vi "leak_tester_0.vi"() -> ()   [LabVIEW 2020]
uses:
  event_controller.ctl
  <vilib>/Spiers New Technologies/SNT/Alfred-Connector/Utilities/Parse Item Label Data Output.ctl
  <vilib>/Spiers New Technologies/SNT/Alfred-Connector/Alfred.lvlib
panel:
  in  "RETURN":bool
  in  "test":bool
  out "Parse Item Label Data out":T1
  out "result":bool
  in  "Barcode":string="IID:287454SN:CM5810B759GBRED11031550695872PN:CM5810B759GBEND"
  out "User ID":string
  out "Enum":T2
  in  "Badge":string="3B 88 01 00 03 08 06 66 00 77 80 78"
  in  "enter":bool
  in  "stop":bool
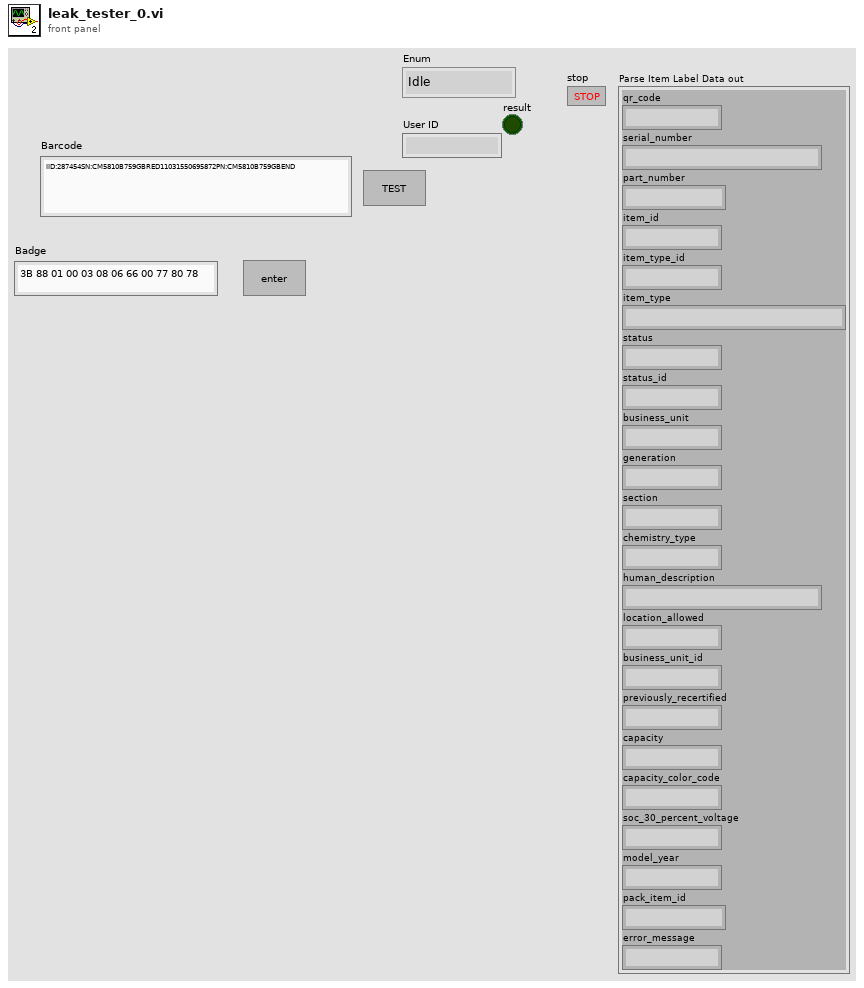
[diagram p1: front panel]
types:
  T1 = typedef "Alfred.lvlib/Parse Item Label Data Output.ctl" = cluster{"qr_code":string, "serial_number":string, "part_number":string, "item_id":string, "item_type_id":string, "item_type":string, "status":string, "status_id":string, "business_unit":string, "generation":string, "section":string, "chemistry_type":string, "human_description":string, "location_allowed":string, "business_unit_id":string, "previously_recertified":string, "capacity":string, "capacity_color_code":string, "soc_30_percent_voltage":string, "model_year":string, "pack_item_id":string, "error_message":string}
  T2 = typedef "event_controller.ctl" = enum16{"Idle", "LoginFalse", "BatteryScan", "BatteryError", "Testing", "Submission"}
  T3 = cluster{"item_id":string, "item_type_id":string, string}
  T4 = cluster{"Username":string, "Badge":string, "Username":string, "Privilege":string}
  T5 = typedef "Alfred.lvlib/Login Info Return.ctl" = cluster{"User ID":string, "Username":string, "First Name":string, "Last Name":string, "E-mail":string, "Time Zone":string, "Error Message":string}
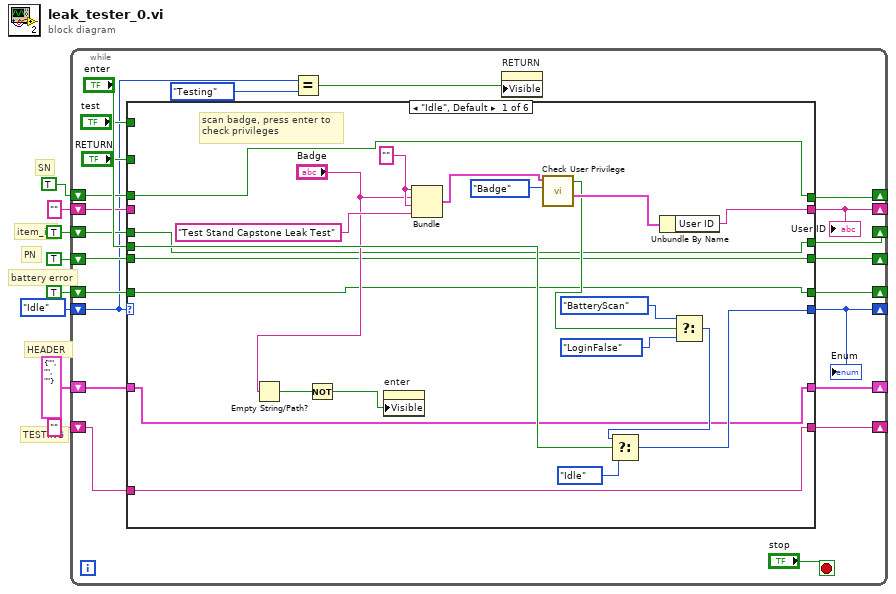
[diagram p0: block diagram]
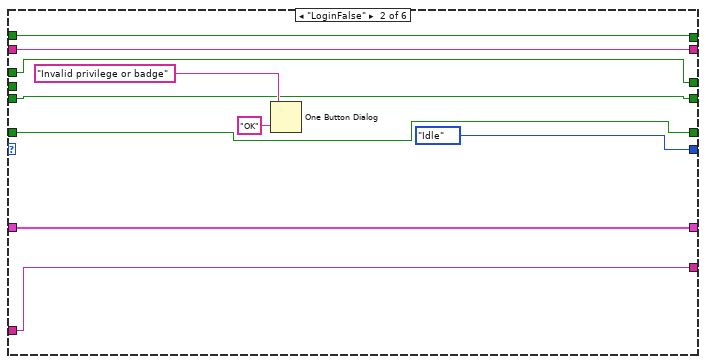
[diagram p2: hidden frame]
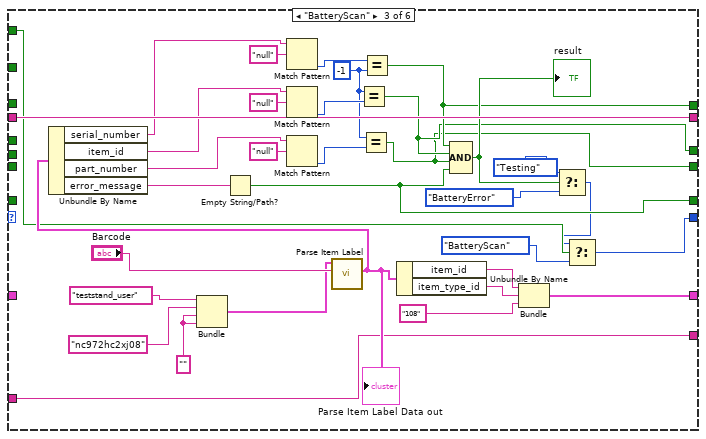
[diagram p3: hidden frame]
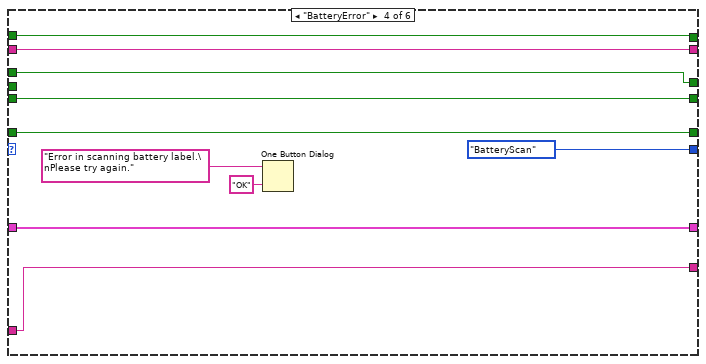
[diagram p4: hidden frame]
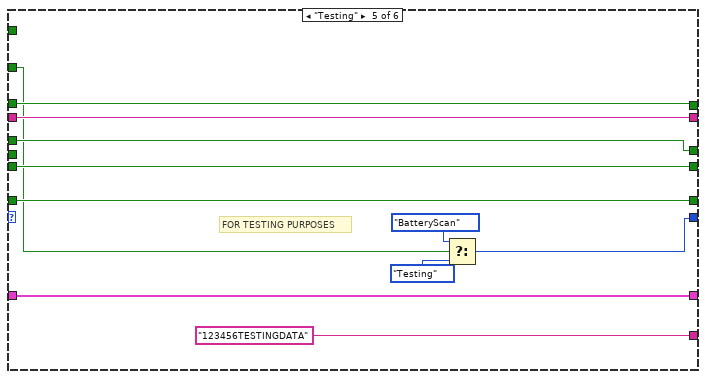
[diagram p5: hidden frame]
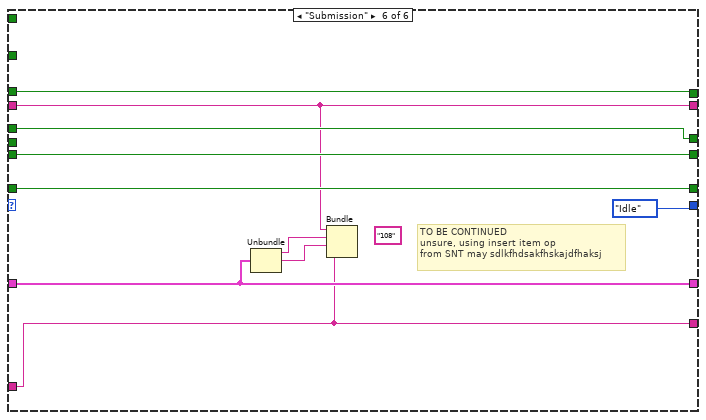
[diagram p6: hidden frame]
diagram:
  # "HEADER"
  # "TESTING"
  # "battery error"
  # "PN"
  # "item_id"
  # "SN"
  n1 = while {
    shift-right: [w29] -> _
    shift-left: event_controller."Idle" -> [w13]
    shift-right: [w27] -> _
    shift-left: "" ("User ID") -> [w26]
    shift-right: [w25] -> _
    shift-left: T3 {"item_id"="", "item_type_id"="", ""} -> [w24]
    shift-right: [w23] -> _
    shift-left: TRUE -> [w22]
    shift-right: [w21] -> _
    shift-left: TRUE -> [w18]
    shift-right: [w20] -> _
    shift-left: TRUE -> [w17]
    shift-right: [w19] -> _
    shift-left: TRUE -> [w16]
    shift-right: [w10] -> _
    shift-left: "" -> [w9]
    stop <- "stop" stop-if-true
    n2 = case shown="\"Idle\", Default" w13 {
      tunnel: [w43 event_controller."Idle" w64 event_controller."BatteryScan" w108 event_controller."Idle"] -> w29
      tunnel: "enter" -> [w44 _ _ _ _ _]
      tunnel: [w40 w59 w96 w106 w117 w122] -> w27
      tunnel: w26 -> [_ w59 w96 w106 w117 w122]
      tunnel: [w36 w58 w87 w105 w116 w121] -> w25
      tunnel: w24 -> [w36 w58 _ w105 w116 w121]
      tunnel: [w35 w57 w71 w104 w115 w126] -> w23
      tunnel: w22 -> [w35 w57 _ w104 w115 w126]
      tunnel: [w34 w56 w70 w103 w114 w125] -> w21
      tunnel: [w33 w55 w69 w102 w113 w124] -> w20
      tunnel: [w32 w54 w68 w101 w112 w123] -> w19
      tunnel: w18 -> [w34 w56 _ w103 w114 w125]
      tunnel: w17 -> [w33 w55 _ w102 w113 w124]
      tunnel: w16 -> [w32 w54 _ w101 w112 w123]
      tunnel: "test" -> [_ _ w67 _ _ _]
      tunnel: "RETURN" -> [_ _ _ _ w111 _]
      tunnel: [w31 w53 w63 w97 "123456TESTINGDATA" w118] -> w10
      tunnel: w9 -> [w31 w53 w63 w97 _ w118]
      frame "Idle", Default {
        w50 = "" ("Username")
        # "scan badge, press enter to \ncheck privileges"
        n3 = Empty String/Path?(string/path="Badge") -> (empty?=w38:bool)
        n4 = Not(x=w38) -> (.not. x?=w37:bool)
        n5 = property on="enter" class="Bool"("Visible"=w37) -> ()  [unwired: 2 in, 2 out]
        n6 = Bundle("Username"=w50, "Badge"="Badge", "Username"=w50, "Privilege"="Test Stand Capstone Leak Test") -> (w48:T4)  [unwired: 1 in]
        n7 = call <vilib>:"Check User Privilege.vi"("Login Method"=enum16{"User ID/PW", "Badge"}."Badge", "Login Data Input"=w48) -> ("Login Info"=w51:T5, "Valid?"=w41:bool)  [unwired: 7 in, 1 out]
        n8 = Unbundle By Name(w51) -> ("User ID"=w40:string)
        n9 = Select(t=event_controller."BatteryScan", s=w41, f=event_controller."LoginFalse") -> (s? t:f=w42:T2)
        n10 = Select(t=w42, s=w44, f=event_controller."Idle") -> (s? t:f=w43:T2)
      }
      frame "LoginFalse" {
        n11 = One Button Dialog(message="Invalid privilege or badge", button name ("OK")="OK") -> ()  [unwired: 1 out]
      }
      frame "BatteryScan" {
        w77 = -1 ("y")
        w93 = ""
        n12 = Bundle("teststand_user", "nc972hc2xj08", w93, w93) -> (w94:cluster{string, string, string, string})  [unwired: 1 in]
        n13 = call <vilib>:"Parse Item Label.vi"("Barcode"="Barcode", "Alfred Data"=w94) -> ("Parse Item Label Data out"=w86:T1)  [unwired: 6 in, 3 out]
        "Parse Item Label Data out" <- w86
        n14 = Unbundle By Name(w86) -> ("serial_number"=w82:string, "item_id"=w81:string, "part_number"=w80:string, "error_message"=w75:string)
        n15 = Empty String/Path?(string/path=w75) -> (empty?=w68:bool)
        n16 = Match Pattern(string=w82, regular expression="null") -> (offset past match=w79:i32)  [unwired: 1 in, 3 out]
        n17 = Match Pattern(string=w81, regular expression="null") -> (offset past match=w78:i32)  [unwired: 1 in, 3 out]
        n18 = Match Pattern(string=w80, regular expression="null") -> (offset past match=w76:i32)  [unwired: 1 in, 3 out]
        n19 = Equal?(x=w77, y=w78) -> (x = y?=w70:bool)
        n20 = Equal?(x=w77, y=w76) -> (x = y?=w69:bool)
        n21 = Equal?(x=w79, y=w77) -> (x = y?=w71:bool)
        n22 = Unbundle By Name(w86) -> ("item_id"=w90:string, "item_type_id"=w89:string)
        n23 = Compound Arithmetic op=AND(w71, w70, w69, w68) -> (w74:bool)
        "result" <- w74
        n24 = Bundle("item_id"=w90, "item_type_id"=w89, "108") -> (w87:T3)  [unwired: 1 in]
        n25 = Select(t=event_controller."Testing", s=w74, f=event_controller."BatteryError") -> (s? t:f=w65:T2)
        n26 = Select(t=w65, s=w67, f=event_controller."BatteryScan") -> (s? t:f=w64:T2)
      }
      frame "BatteryError" {
        n27 = One Button Dialog(message="Error in scanning battery label.\nPlease try again.", button name ("OK")="OK") -> ()  [unwired: 1 out]
      }
      frame "Testing" {
        # "FOR TESTING PURPOSES"
        n28 = Select(t=event_controller."BatteryScan", s=w111, f=event_controller."Testing") -> (s? t:f=w108:T2)
      }
      frame "Submission" {
        (unwired) "108" ("Item Operation ID")
        # "TO BE CONTINUED\nunsure, using insert item op\nfrom SNT may sdlkfhdsakfhskajdfhaksj"
        n29 = Unbundle(w121) -> ("item_id"=w120:string, "item_type_id"=w119:string)  [unwired: 1 out]
        n30 = Bundle("User ID"=w122, "item_id"=w120, "item_type_id"=w119, w118) -> ()  [unwired: 1 in, 1 out]
      }
    }
    "Enum" <- w29
    "User ID" <- w27
    n31 = Equal?(x=w13, y=event_controller."Testing") -> (x = y?=w11:bool)
    n32 = property on="RETURN" class="Bool"("Visible"=w11) -> ()  [unwired: 2 in, 2 out]
  }
